vi "initialize Session Data.vi"(0 "OBJ - Session in":refnum<class "Data DVR Session.lvclass">, 11 "error in":errorcluster) -> (4 "OBJ - Session out":refnum<class "Data DVR Session.lvclass">, 15 "error out":errorcluster)   [LabVIEW 2015, in "Data DVR Session.lvclass"]
doc: "OVERRIDE VI\nPlaceholder for decendant sessions to initialize and set their default values"
uses:
  Data DVR Session.lvclass
  Data DVR Session.lvclass/Data DVR Session.ctl
  Data/Data.lvclass
  Read Data.vi
  Write DVR.vi
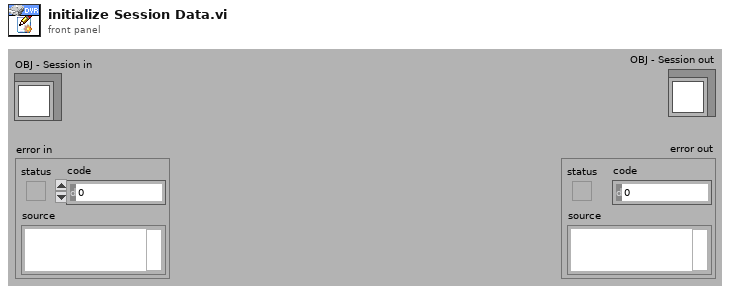
[diagram p1: front panel]
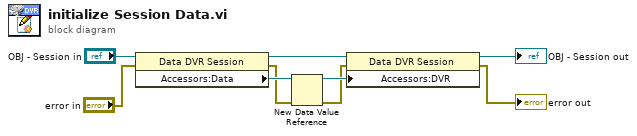
[diagram p0: block diagram]
diagram:
  n1 = property class="Data DVR Session"(reference="OBJ - Session in", error in="error in") -> (reference out=w8:refnum<class "Data DVR Session.lvclass">, error out=w4:errorcluster, "Accessors:Data"=w7:refnum<class "Data.lvclass">)
  n2 = New Data Value Reference(data value=w7, error in=w4) -> (data value reference=w6:refnum<data-value>, error out=w3:errorcluster)
  n3 = property class="Data DVR Session"(reference=w8, error in=w3, "Accessors:DVR"=w6) -> (reference out=→"OBJ - Session out":refnum<class "Data DVR Session.lvclass">, error out=→"error out":errorcluster)
